vi "FTW-Actor-Log-FrameworkEvent.vi"(0 "FTW Actor Instance":refnum<class "FTW-ActorInstance.lvclass">, 5 "Framework Event":T1(ring), 7 "Event Data":string, 11 "error in":errorcluster) -> (4 "FTW Actor Instance out":refnum<class "FTW-ActorInstance.lvclass">, 15 "error out":errorcluster)   [LabVIEW 2012, in "FTW-Actor.lvlib" / "FTW-ActorInstance.lvclass"]
uses:
  FTW-ActorInstance.lvclass
panel:
  # "Inputs"
  # "Outputs"
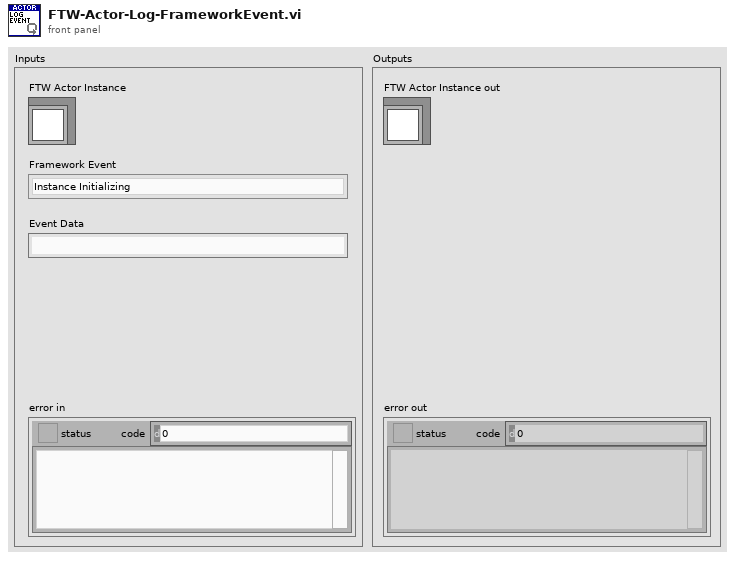
[diagram p1: front panel]
types:
  T1 = enum16{"Instance Initializing", "Instance Initialized", "Instance Job", "Instance Handle Request", "Instance Shutting Down", "Instance Destroyed"}
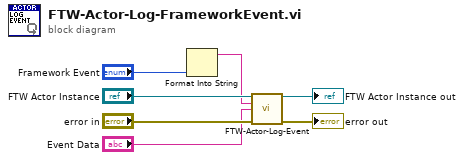
[diagram p0: block diagram]
diagram:
  n1 = Format Into String("Framework Event") -> (resulting string=w1:string)  [unwired: 3 in, 1 out]
  n2 = call-dynamic "FTW-Actor-Log-Event.vi"("Featherweight Actor"="FTW Actor Instance", "Event Type"=w1, "Event Data"="Event Data", "error in"="error in") -> ("Featherweight Actor out"=→"FTW Actor Instance out":refnum<class "FTW-ActorInstance.lvclass">, "error out"=→"error out":errorcluster)  [unwired: 9 in, 1 out]
